vi "Best fit axis-aligned ellipse 2.vi"(0 "x array":dbl[](array[numeric]), 1 "y array":dbl[](array[numeric])) -> (2 "x centre":dbl, 3 "y centre":dbl, 4 "x radius":dbl, 5 "y radius":dbl)   [LabVIEW 2014]
doc: "Finds the best fit axis-aligned ellipse using the Gauss-Newton non-linear least squares method. Input arrays (corresponding values of x and y) must have a minimum of 4 values each"
uses:
  <vilib>/Analysis/baseanly.llb/Real A x B.vi
  <vilib>/Analysis/baseanly.llb/A x Vector.vi
  <vilib>/Analysis/baseanly.llb/Real Inverse Matrix.vi
  <vilib>/Analysis/Matrix/Numeric/Conversions/Array To Matrix - RA2.vi
  <vilib>/Analysis/NI_AALBase.lvlib
  <vilib>/Analysis/Matrix/NI_Matrix.lvlib
panel:
  out "Iters":i32
  # "Paul Nathan 24/06/2015"
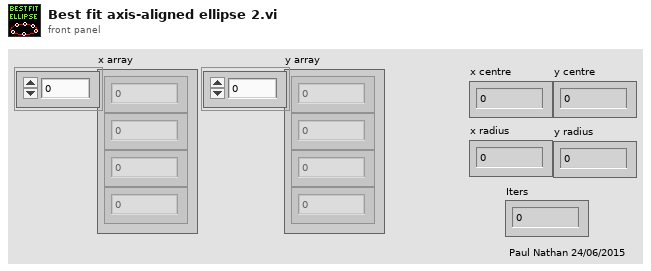
[diagram p1: front panel]
types:
  T1 = typedef "NI_Matrix.lvlib/RealMatrix.ctl" = dbl[][]
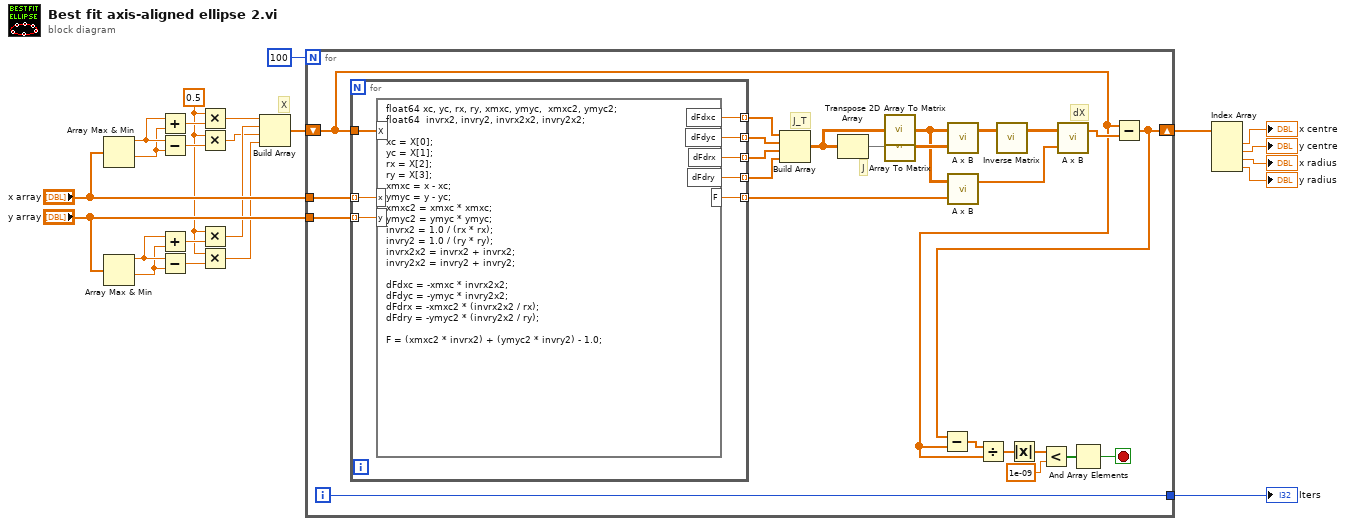
[diagram p0: block diagram]
diagram:
  w13 = 0.5 ("x")
  # "X"
  n1 = Array Max & Min(array="x array") -> (max value=w21:dbl, min value=w20:dbl)  [unwired: 2 out]
  n2 = Array Max & Min(array="y array") -> (max value=w19:dbl, min value=w18:dbl)  [unwired: 2 out]
  n3 = Add(x=w21, y=w20) -> (x+y=w17:dbl)
  n4 = Subtract(x=w21, y=w20) -> (x-y=w16:dbl)
  n5 = Add(x=w19, y=w18) -> (x+y=w14:dbl)
  n6 = Subtract(x=w19, y=w18) -> (x-y=w15:dbl)
  n7 = Multiply(x=w13, y=w17) -> (x*y=w12:dbl)
  n8 = Multiply(x=w13, y=w16) -> (x*y=w10:dbl)
  n9 = Multiply(x=w13, y=w14) -> (x*y=w11:dbl)
  n10 = Multiply(x=w13, y=w15) -> (x*y=w9:dbl)
  n11 = Build Array(w12, w11, w10, w9) -> (w8:dbl[])
  n12 = for {
    N: 100 -> [_]
    tunnel: "x array" -> [w47]
    tunnel: "y array" -> [w46]
    shift-right: [w24] -> w5
    shift-left: w8 -> [w25]
    tunnel: [w32] -> w6
    i -> [w32]
    stop <- w26 stop-if-true
    # "dX"
    # "J_T"
    # "J"
    n13 = for {
      tunnel: w47 -> [w55] mode=indexing
      tunnel: w46 -> [w54] mode=indexing
      tunnel: [w53] -> w45 mode=indexing
      tunnel: [w52] -> w44 mode=indexing
      tunnel: [w51] -> w43 mode=indexing
      tunnel: [w50] -> w42 mode=indexing
      tunnel: [w49] -> w35 mode=indexing
      tunnel: w25 -> [w48]
      n14 = formula code="float64 xc, yc, rx, ry, xmxc, ymyc,  xmxc2, ymyc2;\nfloat64  invrx2, invry2, invrx2x2, invry2x2;\n\nxc = X[0];\nyc = X[1];\nrx = X[2];\nry = X[3];\nxmxc = x - xc;\nymyc = y - yc;\nxmxc2 = xmxc * xmxc;\nymyc2 = ymyc * ymyc;\ninvrx2 = 1.0 / (rx * rx);\ninvry2 = 1.0 / (ry * ry);\ninvrx2x2 = invrx2 + invrx2;\ninvry2x2 = invry2 + invry2;\n\ndFdxc = -xmxc * invrx2x2;\ndFdyc = -ymyc * invry2x2;\ndFdrx = -xmxc2 * (invrx2x2 / rx);\ndFdry = -ymyc2 * (invry2x2 / ry);\n\nF = (xmxc2 * invrx2) + (ymyc2 * invry2) - 1.0;"("x"=w55, "y"=w54, "X"=w48) -> ("dFdxc"=w53:dbl, "dFdyc"=w52:dbl, "dFdrx"=w51:dbl, "dFdry"=w50:dbl, "F"=w49:dbl)
    }
    n15 = Build Array(w45, w44, w43, w42) -> (w37:dbl[][])
    n16 = Transpose 2D Array(2D array=w37) -> (transposed array=w41:dbl[][])
    n17 = call-poly <vilib>:"Array To Matrix.vi"("Real 2D Array"=w37) -> ("Real Matrix"=w36:T1)
    n18 = call-poly <vilib>:"Array To Matrix.vi"("Real 2D Array"=w41) -> ("Real Matrix"=w40:T1)
    n19 = call-poly <vilib>:"A x B.vi"("B"=w40, "A"=w36) -> ("A x B"=w39:T1)  [unwired: 1 out]
    n20 = call-poly <vilib>:"A x B.vi"("Vector"=w35, "A"=w36) -> ("A x Vector"=w34:dbl[])  [unwired: 1 out]
    n21 = call-poly <vilib>:"Inverse Matrix.vi"("Input Matrix"=w39) -> ("Inverse Matrix"=w38:T1)  [unwired: 1 in, 1 out]
    n22 = call-poly <vilib>:"A x B.vi"("Vector"=w34, "A"=w38) -> ("A x Vector"=w33:dbl[])  [unwired: 1 out]
    n23 = Subtract(x=w25, y=w33) -> (x-y=w24:dbl[])
    n24 = Subtract(x=w24, y=w25) -> (x-y=w31:dbl[])
    n25 = Divide(x=w31, y=w25) -> (x/y=w30:dbl[])
    n26 = Absolute Value(x=w30) -> (abs(x)=w29:dbl[])
    n27 = Less?(x=w29, y=1e-09) -> (x < y?=w27:bool[])
    n28 = And Array Elements(Boolean array=w27) -> (logical AND=w26:bool)
  }
  "Iters" <- w6
  n29 = Index Array(array=w5) -> (element #1=→"x centre":dbl, element #2=→"y centre":dbl, element #3=→"x radius":dbl, element #4=→"y radius":dbl)  [unwired: 4 in]
